vi "Sub Super Duper_2014 06 25_JWa.vi"(0 "VISA resource name":refnum<visa-resource-name>="GPIB0::17::INSTR", 1 "Sample Properties:":T9 {"Date Created" format="%<%Y/%m/%d>T"}, 2 "Gated SMU4 is...":bool, 3 "TRF Cluster":T10={"Step 4"=-38.0, "# of Loops"=1.0, "Transfer 2"=FALSE, "Start 4"=-2.0, "Total Points 2"=2, "Start 3"=40.0, "Stop 2"=-40.0, "Step 3"=-1.0, "Loop Step"=0.0, "Integration Time 3"=0, "Loop Wait"=0.0, "First Step"=0.0} {"Loop Wait" format="%<%H:%M:%S>t"; "Integration Time 3" scale=0.0..2.0; "Step 3" format="%.2f"; "Stop 2" format="%.2f"; "Start 3" format="%.2f"; "Start 4" format="%.2f"; "Step 4" format="%.2f"}, 4 "TSP Cluster":T11={"Transport"=FALSE, "Start 2"=0.0, "Stop 3"=-60.0, "Step 2"=-1.0, "Start"=0.0, "Step"=-10.0, "Total Points"=7, "Integration Time"=0} {"Integration Time" scale=0.0..2.0; "Step" format="%.2f"; "Start" format="%.2f"; "Step 2" format="%.2f"; "Stop 3" format="%.2f"; "Start 2" format="%.2f"}, 5 "Compliance Cluster":T6={"Var1 sweep settings"={"sweep spacing (linear: 0)"=0, "sweep mode"=FALSE, "compliance (V)"=100.0, "compliance (A)"=0.001}, "Var1 sweep settings 2"={"sweep spacing (linear: 0)"=0, "sweep mode"=FALSE, "compliance (V)"=100.0, "compliance (A)"=0.001}, "Var2 step settings 2"={"compliance (A)"=0.001, "compliance (V)"=100.0}, "Var2 step settings"={"compliance (A)"=0.001, "compliance (V)"=100.0}} {"Var2 step settings"."compliance (V)" format="%.2f"; "Var2 step settings"."compliance (A)" format="%^.2e"; "Var2 step settings 2"."compliance (V)" format="%.2f"; "Var2 step settings 2"."compliance (A)" format="%^.2e"; "Var1 sweep settings 2"."compliance (A)" format="%^.2e"; "Var1 sweep settings 2"."compliance (V)" format="%.2f"; "Var1 sweep settings 2"."sweep spacing (linear: 0)" items=["linear", "log 10", "log 25", "log 50"]; "Var1 sweep settings"."compliance (A)" format="%^.2e"; "Var1 sweep settings"."compliance (V)" format="%.2f"; "Var1 sweep settings"."sweep spacing (linear: 0)" items=["linear", "log 10", "log 25", "log 50"]}, 6 "Light Bathe Cluster":T2={"TG to BG:  "=FALSE, "TG to BG Durration"=120.0, "TRF to TSP:   "=FALSE, "TRF to TSP Duration"=120.0, "Post Measure: "=FALSE, "TG to BG (TSP):"=FALSE, "TG to BG Durration 3"=120.0} {"TG to BG Durration 3" format="%<%H:%M:%S>t"; "TRF to TSP Duration" format="%<%H:%M:%S>t"; "TG to BG Durration" format="%<%H:%M:%S>t"}, 7 "error in":errorcluster, 8 "Saved Folder:":path=path "C:/1DATA/2011", 9 "Wait Cluster":T5 {"Wait Time (s)" format="%.1g"; "Wait Countdown" format="%<%H:%M:%S%1u>t"}, 10 "Ambient Temp (Y/N)":bool=TRUE, 11 "TG Dielectric Prop":T1, 15 "Loop Count":dbl, 16 "Gate Current Cluster":T3={"Gate Current (TSP)"={"Y2 axis on/off"=FALSE, "MINIMUM"=0.0, "MAXIMUM"=1.0, "Variable name"="Ig", "LIN or LOG axis"="LIN"}, "Gate Current (TRF)"={"Y2 axis on/off"=FALSE, "MINIMUM"=0.0, "MAXIMUM"=1.0, "Variable name"="Ig", "LIN or LOG axis"="LIN"}} {"Gate Current (TSP)"."MAXIMUM" format="%.9f"; "Gate Current (TSP)"."MINIMUM" format="%.9f"; "Gate Current (TRF)"."MAXIMUM" format="%.9f"; "Gate Current (TRF)"."MINIMUM" format="%.9f"}, 17 "Dielectric Constant (BG)":dbl) -> (12 "Status Indicator":bool, 14 "Vt Cluster":T4 {"Id Max" format="%.3g"; "Vt Max" format="%.3g"; "Vt Min" format="%.3g"; "Vt Ratio" format="%.3g"}, 20 "VISA resource name out":refnum<visa-resource-name>, 21 "TRF Path":path, 23 "TSP Path":path, 24 "Graph Cluster":T7, 25 "Char Cluster":T8 {"Mobility-Lin" format="%#_4e"; "On/Off" format="%#_4e"; "Mobility-Sat" format="%#_4e"}, 27 "error out":errorcluster)   [LabVIEW 2012]
panel:
  out "LKG Path":path
  # "Vg Sweep"
  # "Vd Step"
  # "Loops and Integration Time"
  # "Device Characteristics"
  # "Light Bath is..."
  # "Duration (hh:mm:ss)"
  # "Sample Properties:"
  # "%"
  # "nm"
  # "Device Properties:"
  # "um"
  # "um"
  # "Vg Step"
  # "Vd Step"
  # "Integration Time"
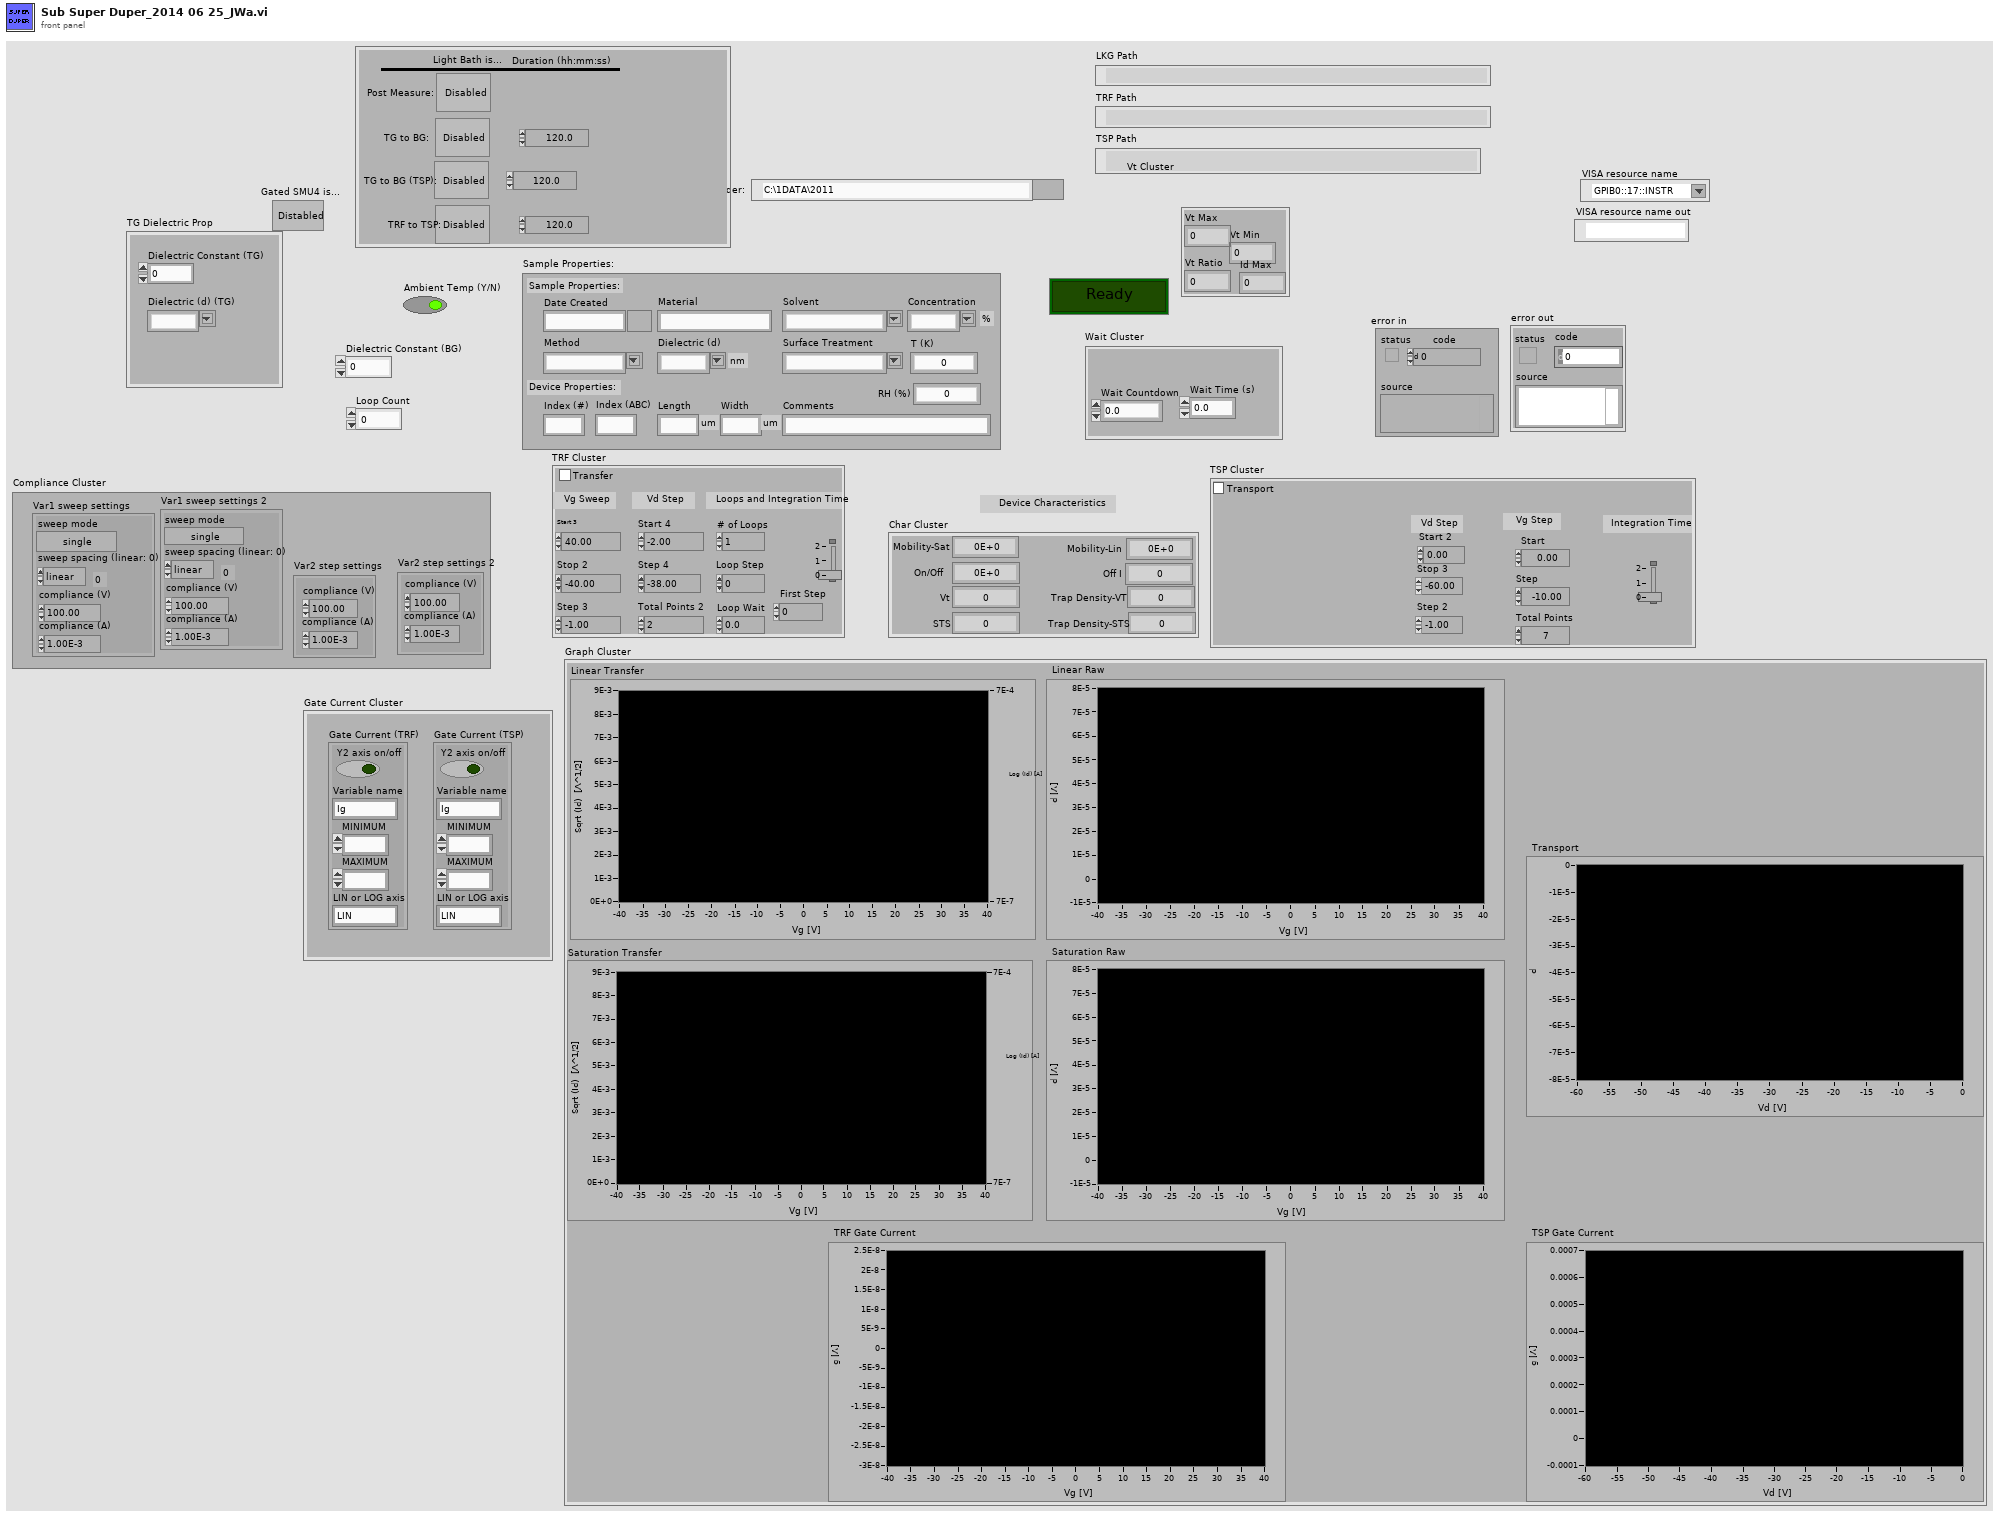
[diagram p1: front panel]
types:
  T1 = cluster{"Dielectric Constant (TG)":dbl, "Dielectric (d) (TG)":string}
  T2 = cluster{"TG to BG:  ":bool, "TG to BG Durration":dbl, "TRF to TSP:   ":bool, "TRF to TSP Duration":dbl, "Post Measure: ":bool, "TG to BG (TSP):":bool, "TG to BG Durration 3":dbl}
  T3 = cluster{"Gate Current (TSP)":cluster{"Y2 axis on/off":bool, "MINIMUM":ext, "MAXIMUM":ext, "Variable name":string, "LIN or LOG axis":string}, "Gate Current (TRF)":cluster{"Y2 axis on/off":bool, "MINIMUM":ext, "MAXIMUM":ext, "Variable name":string, "LIN or LOG axis":string}}
  T4 = cluster{"Vt Max":i32, "Vt Min":i32, "Vt Ratio":i32, "Id Max":i32}
  T5 = cluster{"Wait Countdown":dbl, "Wait Time (s)":dbl}
  T6 = cluster{"Var1 sweep settings":cluster{"sweep spacing (linear: 0)":u16, "sweep mode":bool, "compliance (V)":dbl, "compliance (A)":dbl}, "Var1 sweep settings 2":cluster{"sweep spacing (linear: 0)":u16, "sweep mode":bool, "compliance (V)":dbl, "compliance (A)":dbl}, "Var2 step settings 2":cluster{"compliance (A)":dbl, "compliance (V)":dbl}, "Var2 step settings":cluster{"compliance (A)":dbl, "compliance (V)":dbl}}
  T7 = cluster{"Linear Transfer":cluster{dbl[], "trace":dbl[]}[], "Linear Raw":cluster{dbl[], dbl[]}[], "Saturation Transfer":cluster{dbl[], "trace":dbl[]}[], "Saturation Raw":cluster{dbl[], dbl[]}[], "Transport":cluster{dbl[], dbl[]}[], "TRF Gate Current":cluster{dbl[], dbl[]}[], "TSP Gate Current":cluster{dbl[], dbl[]}[]}
  T8 = cluster{"Mobility-Sat":dbl, "Mobility-Lin":dbl, "On/Off ":dbl, "Off I":dbl, "Vt":dbl, "STS":dbl, "Trap Density-VT":dbl, "Trap Density-STS":dbl}
  T9 = cluster{"Date Created":timestamp, "Material":string, "Solvent":string, "Concentration":string, "Method":string, "Dielectric (d)":string, "Index (#)":string, "Index (ABC)":string, "Length":string, "Width":string, "Surface Treatment":string, "Comments":string, "T (K)":dbl, "RH (%)":dbl}
  T10 = cluster{"Step 4":dbl, "# of Loops":dbl, "Transfer 2":bool, "Start 4":dbl, "Total Points 2":u16, "Start 3":dbl, "Stop 2":dbl, "Step 3":dbl, "Loop Step":dbl, "Integration Time 3":u32, "Loop Wait":dbl, "First Step":dbl}
  T11 = cluster{"Transport":bool, "Start 2":dbl, "Stop 3":dbl, "Step 2":dbl, "Start":dbl, "Step":dbl, "Total Points":u16, "Integration Time":u32}
  T12 = cluster{"Vname":string, "Vname 2":string, "Vname 3":string, "Vname 4":string, "Iname":string, "Iname 2":string, "Iname 3":string, "Iname 4":string, "Mode":u16, "Mode 2":u16, "Mode 3":u16, "Mode 4":u16, "Function":u16, "Function 2":u16, "Function 3":u16, "Function 4":u16, "Value (V or A)":dbl, "Value (Either V or A) 2":dbl, "Value (Either V or A) 3":dbl, "Value (Either V or A) 4":dbl}
  T13 = cluster{"Vt Max":i32, "Vt Min":i32, "Vt Ratio":i32, "Id Max":dbl}
  T14 = cluster{"Mobility-Sat":dbl, "Mobility-Lin":dbl, "On/Off Current":dbl, "Off I":dbl, "Vt":dbl, "STS":dbl, "Trap Density-VT":dbl, "Trap Density-STS":dbl}
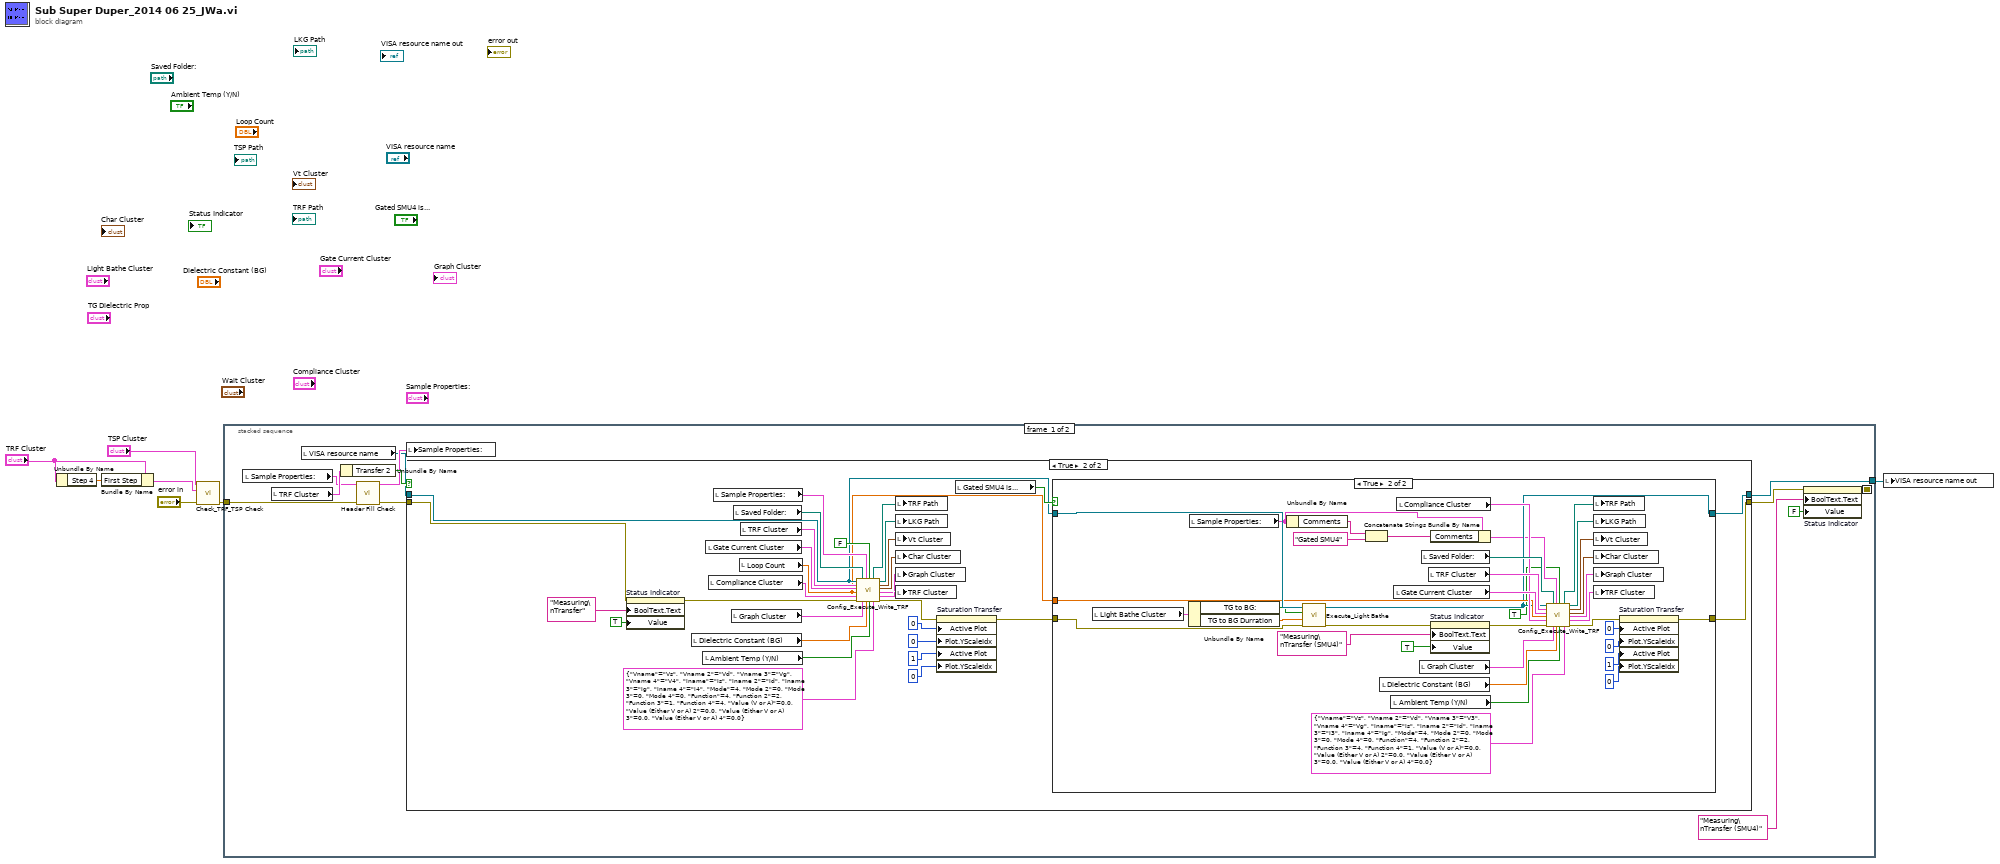
[diagram p0: block diagram]
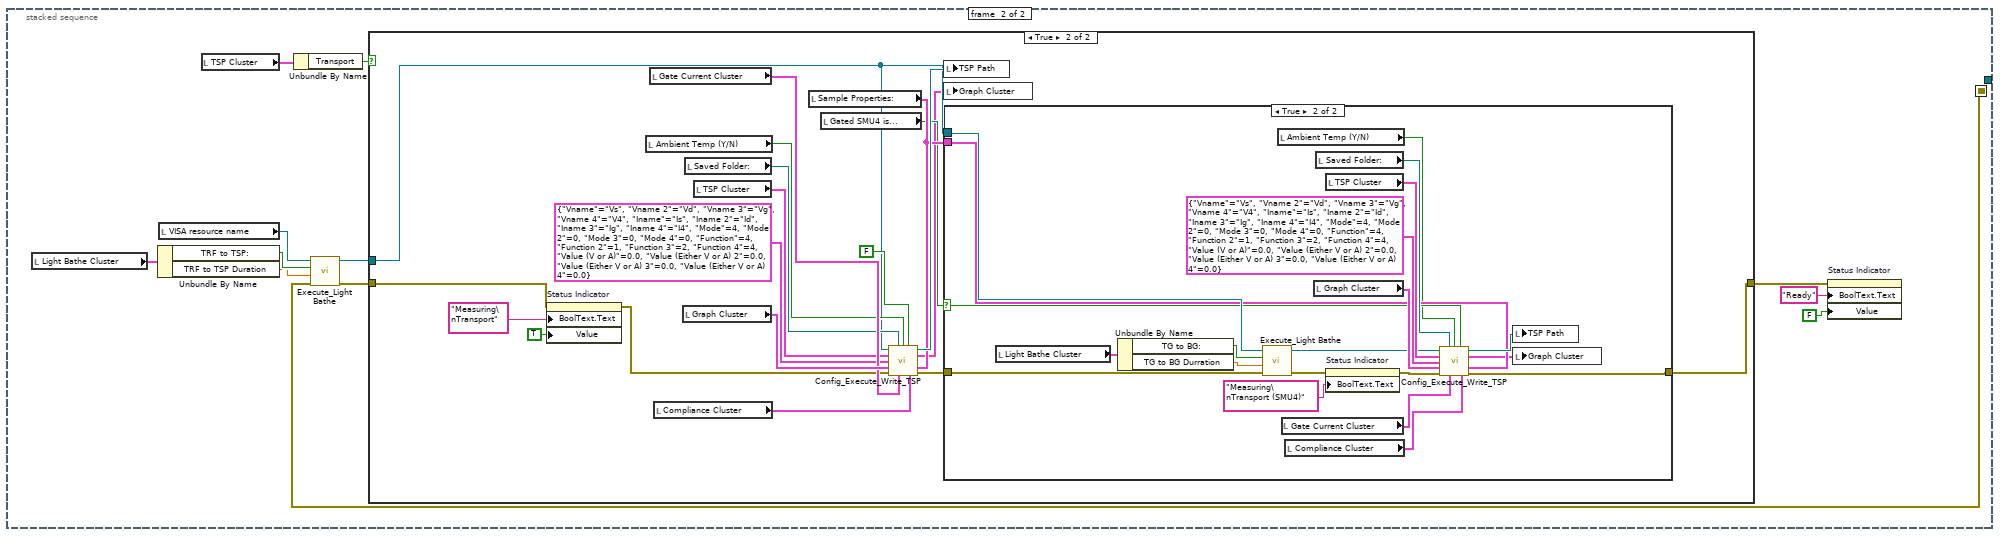
[diagram p4: hidden frame]
diagram:
  n1 = Unbundle By Name("TRF Cluster") -> ("Step 4"=w6:dbl)
  n2 = Bundle By Name(cluster="TRF Cluster", "First Step"=w6) -> (w2:T10)
  n3 = call "Check_TRF_TSP Check.vi"("error in"="error in", "TRF Cluster"=w2, "TSP Cluster"="TSP Cluster") -> ("error out"=w3:errorcluster)  [unwired: 8 in]
  n4 = stacked-sequence {
    seq-local: [w8 _] -> [_ w94]
    tunnel: [w17 _] -> w5
    tunnel: w3 -> [w11 _]
    frame #0 {
      n5 = local read "Sample Properties:"() -> (w13:T9)
      n6 = local read "TRF Cluster"() -> (w18:T10)
      n7 = local read "VISA resource name"() -> (w9:refnum<visa-resource-name>)
      n8 = Unbundle By Name(w18) -> ("Transfer 2"=w19:bool)
      n9 = call "Header Fill Check.vi"("error in (no error)"=w11, "Sample Properties:"=w13) -> ("error out"=w10:errorcluster, "Cluster"=w12:T9)  [unwired: 8 in]
      n10 = local write "Sample Properties:"(w12) -> ()
      n11 = case shown="True" w19 {
        tunnel: [w20 w52] -> w17
        tunnel: w10 -> [w21 w51]
        tunnel: [w21 w24] -> w14
        tunnel: w9 -> [w20 w23]
        frame False {
        }
        frame True {
          n12 = property on="Status Indicator" class="Bool (strict)"(error in=w51, "BoolText.Text"="Measuring\nTransfer", "Value"=TRUE) -> (error out=w30:errorcluster)  [unwired: 1 in, 1 out]
          n13 = local read "Dielectric Constant (BG)"() -> (w38:dbl)
          n14 = local read "Ambient Temp (Y/N)"() -> (w25:bool)
          n15 = local read "Gate Current Cluster"() -> (w39:T3)
          n16 = local read "Compliance Cluster"() -> (w45:T6)
          n17 = local read "Sample Properties:"() -> (w36:T9)
          n18 = local read "Graph Cluster"() -> (w41:T7)
          n19 = local read "Saved Folder:"() -> (w37:path)
          n20 = local read "Loop Count"() -> (w22:dbl)
          n21 = local read "TRF Cluster"() -> (w32:T10)
          n22 = call "Config_Execute_Write_TRF.vi"("VISA Refnum in"=w23, "TRF Cluster in"=w32, "Gate Current Cluster"=w39, "Loop Count"=w22, "Compliance Cluster"=w45, "Error In"=w30, "Saved Folder:"=w37, "Graph Cluster"=w41, "Sample Properties:"=w36, "Dielectric Constant (BG)"=w38, "SMU4? (Y/N)"=FALSE, "Ambient Temp (Y/N)"=w25, "SMU Config"=T12 {"Vname"="Vs", "Vname 2"="Vd", "Vname 3"="Vg", "Vname 4"="V4", "Iname"="Is", "Iname 2"="Id", "Iname 3"="Ig", "Iname 4"="I4", "Mode"=4, "Mode 2"=0, "Mode 3"=0, "Mode 4"=0, "Function"=4, "Function 2"=2, "Function 3"=1, "Function 4"=4, "Value (V or A)"=0.0, "Value (Either V or A) 2"=0.0, "Value (Either V or A) 3"=0.0, "Value (Either V or A) 4"=0.0}) -> ("Filepath Out 2"=w35:path, "Filepath Out"=w34:path, "Check Cluster"=w42:T13, "Output"=w43:T14, "Graph Cluster out"=w40:T7, "TRF Cluster out"=w44:T10, "error out"=w33:errorcluster)
          n23 = local write "TRF Path"(w35) -> ()
          n24 = local write "LKG Path"(w34) -> ()
          n25 = local write "Vt Cluster"(w42) -> ()
          n26 = local write "Char Cluster"(w43) -> ()
          n27 = local write "Graph Cluster"(w40) -> ()
          n28 = local write "TRF Cluster"(w44) -> ()
          n29 = property on="Saturation Transfer" class="XYGraph (strict)"(error in=w33, "Active Plot"=0, "Plot.YScaleIdx"=0, "Active Plot"=1, "Plot.YScaleIdx"=0) -> (error out=w29:errorcluster)  [unwired: 1 in, 1 out]
          n30 = local read "Gated SMU4 is..."() -> (w26:bool)
          n31 = case shown="True" w26 {
            tunnel: w29 -> [w53 w91]
            tunnel: w23 -> [w54 w90]
            tunnel: w22 -> [_ w65]
            tunnel: [w54 w64] -> w52
            tunnel: [w53 w59] -> w24
            frame False {
            }
            frame True {
              n32 = local read "Light Bathe Cluster"() -> (w57:T2)
              n33 = Unbundle By Name(w57) -> ("TG to BG:"=w56:bool, "TG to BG Durration"=w55:dbl)
              n34 = local read "Sample Properties:"() -> (w63:T9)
              n35 = Unbundle By Name(w63) -> ("Comments"=w89:string)
              n36 = call "Execute_Light Bathe.vi"("VISA Refnum in"=w90, "Execute?"=w56, "Duration"=w55, "error in (no error)"=w91) -> ("VISA Out"=w64:refnum<visa-resource-name>, "Error Out"=w66:errorcluster)  [unwired: 5 in]
              n37 = Concatenate Strings(w89, "Gated SMU4" ("string")) -> (w87:string)
              n38 = local read "Dielectric Constant (BG)"() -> (w79:dbl)
              n39 = local read "Ambient Temp (Y/N)"() -> (w58:bool)
              n40 = local read "Gate Current Cluster"() -> (w78:T3)
              n41 = local read "Compliance Cluster"() -> (w72:T6)
              n42 = local read "Graph Cluster"() -> (w76:T7)
              n43 = local read "Saved Folder:"() -> (w80:path)
              n44 = local read "TRF Cluster"() -> (w84:T10)
              n45 = Bundle By Name(cluster=w63, "Comments"=w87) -> (w62:T9)
              n46 = property on="Status Indicator" class="Bool (strict)"(error in=w66, "BoolText.Text"="Measuring\nTransfer (SMU4)", "Value"=TRUE) -> (error out=w86:errorcluster)  [unwired: 1 in, 1 out]
              n47 = call "Config_Execute_Write_TRF.vi"("VISA Refnum in"=w64, "TRF Cluster in"=w84, "Gate Current Cluster"=w78, "Loop Count"=w65, "Compliance Cluster"=w72, "Error In"=w86, "Saved Folder:"=w80, "Graph Cluster"=w76, "Sample Properties:"=w62, "Dielectric Constant (BG)"=w79, "SMU4? (Y/N)"=TRUE, "Ambient Temp (Y/N)"=w58, "SMU Config"=T12 {"Vname"="Vs", "Vname 2"="Vd", "Vname 3"="V3", "Vname 4"="Vg", "Iname"="Is", "Iname 2"="Id", "Iname 3"="I3", "Iname 4"="Ig", "Mode"=4, "Mode 2"=0, "Mode 3"=0, "Mode 4"=0, "Function"=4, "Function 2"=2, "Function 3"=4, "Function 4"=1, "Value (V or A)"=0.0, "Value (Either V or A) 2"=0.0, "Value (Either V or A) 3"=0.0, "Value (Either V or A) 4"=0.0}) -> ("Filepath Out 2"=w81:path, "Filepath Out"=w82:path, "Check Cluster"=w75:T13, "Output"=w74:T14, "Graph Cluster out"=w77:T7, "TRF Cluster out"=w73:T10, "error out"=w83:errorcluster)
              n48 = local write "TRF Path"(w81) -> ()
              n49 = local write "LKG Path"(w82) -> ()
              n50 = local write "Vt Cluster"(w75) -> ()
              n51 = local write "Char Cluster"(w74) -> ()
              n52 = local write "Graph Cluster"(w77) -> ()
              n53 = local write "TRF Cluster"(w73) -> ()
              n54 = property on="Saturation Transfer" class="XYGraph (strict)"(error in=w83, "Active Plot"=0, "Plot.YScaleIdx"=0, "Active Plot"=1, "Plot.YScaleIdx"=0) -> (error out=w59:errorcluster)  [unwired: 1 in, 1 out]
            }
          }
        }
      }
      n55 = property on="Status Indicator" class="Bool (strict)"(error in=w14, "BoolText.Text"="Measuring\nTransfer (SMU4)", "Value"=FALSE) -> (error out=w8:errorcluster)  [unwired: 1 in, 1 out]
    }
    frame #1 {
      n56 = local read "Light Bathe Cluster"() -> (w98:T2)
      n57 = Unbundle By Name(w98) -> ("TRF to TSP:"=w96:bool, "TRF to TSP Duration"=w95:dbl)
      n58 = local read "VISA resource name"() -> (w97:refnum<visa-resource-name>)
      n59 = local read "TSP Cluster"() -> (w103:T11)
      n60 = Unbundle By Name(w103) -> ("Transport"=w102:bool)
      n61 = call "Execute_Light Bathe.vi"("VISA Refnum in"=w97, "Execute?"=w96, "Duration"=w95, "error in (no error)"=w94) -> ("VISA Out"=w92:refnum<visa-resource-name>, "Error Out"=w93:errorcluster)  [unwired: 5 in]
      n62 = case shown="True" w102 {
        tunnel: [w104 w108] -> w101
        tunnel: w93 -> [w104 w107]
        tunnel: w92 -> [_ w106]
        frame False {
        }
        frame True {
          n63 = property on="Status Indicator" class="Bool (strict)"(error in=w107, "BoolText.Text"="Measuring\nTransport", "Value"=TRUE) -> (error out=w116:errorcluster)  [unwired: 1 in, 1 out]
          n64 = local read "Ambient Temp (Y/N)"() -> (w111:bool)
          n65 = local read "Gate Current Cluster"() -> (w120:T3)
          n66 = local read "Compliance Cluster"() -> (w122:T6)
          n67 = local read "Graph Cluster"() -> (w121:T7)
          n68 = local read "Saved Folder:"() -> (w119:path)
          n69 = local read "TSP Cluster"() -> (w117:T11)
          n70 = local read "Sample Properties:"() -> (w113:T9)
          n71 = local read "Gated SMU4 is..."() -> (w112:bool)
          n72 = call "Config_Execute_Write_TSP.vi"("VISA Refnum in"=w106, "Saved Folder:"=w119, "Ambient Temp (Y/N)"=w111, "SMU4? (Y/N)"=FALSE, "TSP Cluster"=w117, "SMU Config"=T12 {"Vname"="Vs", "Vname 2"="Vd", "Vname 3"="Vg", "Vname 4"="V4", "Iname"="Is", "Iname 2"="Id", "Iname 3"="Ig", "Iname 4"="I4", "Mode"=4, "Mode 2"=0, "Mode 3"=0, "Mode 4"=0, "Function"=4, "Function 2"=1, "Function 3"=2, "Function 4"=4, "Value (V or A)"=0.0, "Value (Either V or A) 2"=0.0, "Value (Either V or A) 3"=0.0, "Value (Either V or A) 4"=0.0}, "Graph Cluster in"=w121, "Sample Properties:"=w113, "error In"=w116, "Gate Current Cluster"=w120, "Compliance Cluster"=w122) -> ("Filepath Out"=w118:path, "Graph Cluster out"=w105:T7, "error Out"=w115:errorcluster)  [unwired: 2 in]
          n73 = local write "TSP Path"(w118) -> ()
          n74 = local write "Graph Cluster"(w105) -> ()
          n75 = case shown="True" w112 {
            selector: w112 -> [_ w131]
            tunnel: w106 -> [_ w145]
            tunnel: w115 -> [w124 w144]
            tunnel: w113 -> [_ w133]
            tunnel: [w124 w126] -> w108
            frame False {
            }
            frame True {
              n76 = local read "Light Bathe Cluster"() -> (w129:T2)
              n77 = Unbundle By Name(w129) -> ("TG to BG:"=w128:bool, "TG to BG Durration"=w127:dbl)
              n78 = call "Execute_Light Bathe.vi"("VISA Refnum in"=w145, "Execute?"=w128, "Duration"=w127, "error in (no error)"=w144) -> ("VISA Out"=w134:refnum<visa-resource-name>, "Error Out"=w132:errorcluster)  [unwired: 5 in]
              n79 = local read "Ambient Temp (Y/N)"() -> (w130:bool)
              n80 = local read "Gate Current Cluster"() -> (w138:T3)
              n81 = local read "Compliance Cluster"() -> (w136:T6)
              n82 = local read "Graph Cluster"() -> (w137:T7)
              n83 = local read "Saved Folder:"() -> (w139:path)
              n84 = local read "TSP Cluster"() -> (w141:T11)
              n85 = property on="Status Indicator" class="Bool (strict)"(error in=w132, "BoolText.Text"="Measuring\nTransport (SMU4)") -> (error out=w142:errorcluster)  [unwired: 1 in, 1 out]
              n86 = call "Config_Execute_Write_TSP.vi"("VISA Refnum in"=w134, "Saved Folder:"=w139, "Ambient Temp (Y/N)"=w130, "SMU4? (Y/N)"=w131, "TSP Cluster"=w141, "SMU Config"=T12 {"Vname"="Vs", "Vname 2"="Vd", "Vname 3"="Vg", "Vname 4"="V4", "Iname"="Is", "Iname 2"="Id", "Iname 3"="Ig", "Iname 4"="I4", "Mode"=4, "Mode 2"=0, "Mode 3"=0, "Mode 4"=0, "Function"=4, "Function 2"=1, "Function 3"=2, "Function 4"=4, "Value (V or A)"=0.0, "Value (Either V or A) 2"=0.0, "Value (Either V or A) 3"=0.0, "Value (Either V or A) 4"=0.0}, "Graph Cluster in"=w137, "Sample Properties:"=w133, "error In"=w142, "Gate Current Cluster"=w138, "Compliance Cluster"=w136) -> ("Filepath Out"=w140:path, "Graph Cluster out"=w125:T7, "error Out"=w126:errorcluster)  [unwired: 2 in]
              n87 = local write "TSP Path"(w140) -> ()
              n88 = local write "Graph Cluster"(w125) -> ()
            }
          }
        }
      }
      n89 = property on="Status Indicator" class="Bool (strict)"(error in=w101, "BoolText.Text"="Ready", "Value"=FALSE) -> ()  [unwired: 1 in, 2 out]
    }
  }
  n90 = local write "VISA resource name out"(w5) -> ()
